vi "IMAQdx Get Image Data.vi"(7 "Buffer Number Mode (Next)":T1, 8 "error in":errorcluster, 9 "Buffer Number In":u32, 11 "Session In":T2) -> (0 "error out":errorcluster, 1 "Buffer Number Out":u32, 2 "Image Data Array":u8[](array[numeric]), 3 "Session Out":T2)   [LabVIEW 2020, in "NI_Vision_Acquisition_Software.lvlib"]
doc: "Copies the raw data of the specified frame into <B>Image Data Array</B>. Call this VI only after calling the IMAQdx Configure Acquisition VI."
uses:
  NI_Vision_Acquisition_Software.lvlib
  IMAQdx.ctl
  IMAQdx Buffer Number Mode.ctl
  niimaqdx.dll
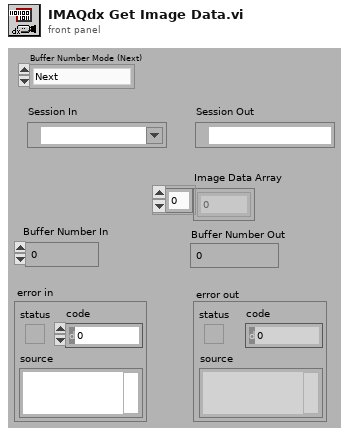
[diagram p1: front panel]
types:
  T1 = typedef "NI_Vision_Acquisition_Software.lvlib/IMAQdx Buffer Number Mode.ctl" = enum32{"Next", "Last", "Buffer Number", "Every", "Last New"}
  T2 = typedef "IMAQdx.ctl" = refnum<k21>
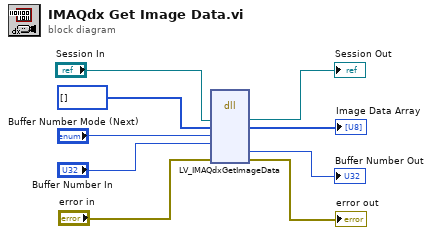
[diagram p0: block diagram]
diagram:
  n1 = dll-call lib="niimaqdx.dll" fn="LV_IMAQdxGetImageData"("Session In"="Session In", "Image Data Array"=u8[] [], "bufferNumberMode"="Buffer Number Mode (Next)", "bufferNumberDesired"="Buffer Number In", "error in"="error in") -> ("Session In"=→"Session Out":T2, "Image Data Array"=→"Image Data Array":u8[], "bufferNumberActual"=→"Buffer Number Out":u32, "error in"=→"error out":errorcluster)  [unwired: 7 in, 2 out]
